vi "Move(SubVI for PI).vi"(5 "Goal":dbl format="%#_13g", 6 "index":i8, 7 "error in":errorcluster) -> (0 "Position After Move":dbl[](array[numeric]) format="%.6f", 3 "error out":errorcluster)   [LabVIEW 2020]
uses:
  Global Parameters.vi
panel:
  out "Position of Global before Move":dbl[](array[numeric])=[95.0] format="%.6f"
  out "Move time":u32
  out "Move+Read Time":u32
  in  "stop":bool
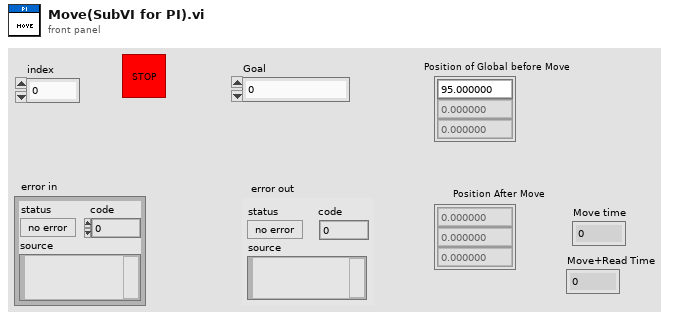
[diagram p1: front panel]
types:
  T1 = enum32{"Bad", "Idle", "Run top level", "Running"}
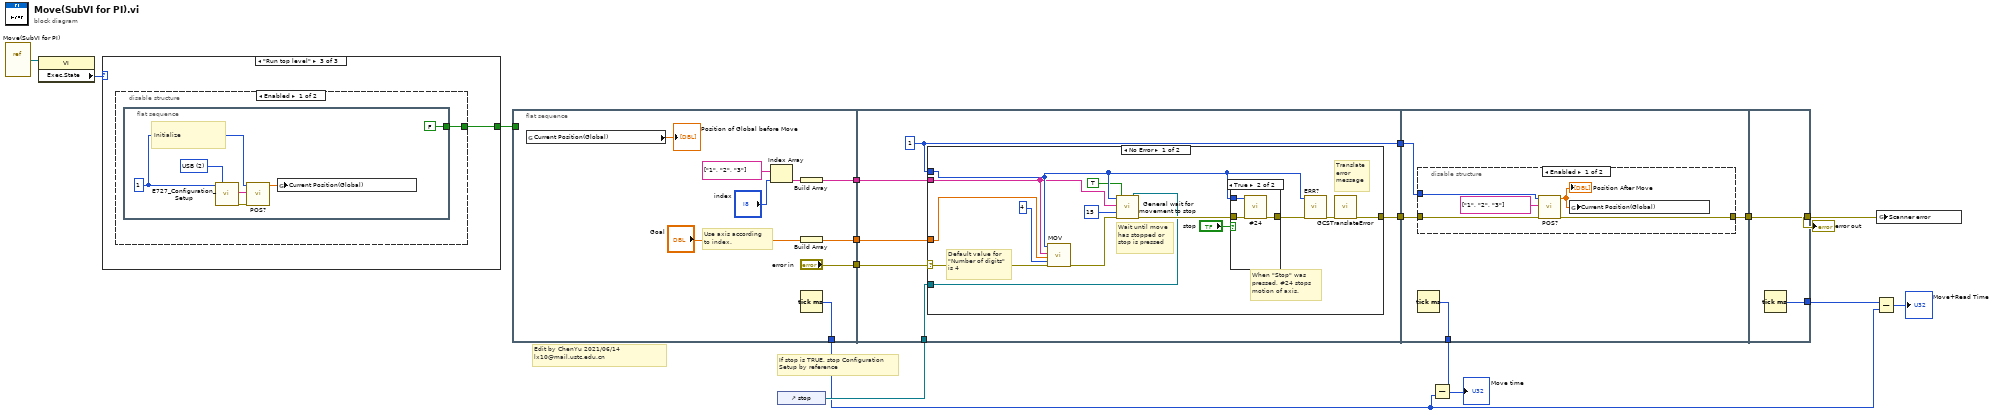
[diagram p0: block diagram]
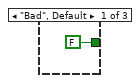
[diagram p2: hidden frame]
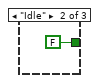
[diagram p3: hidden frame]
diagram:
  # "Edit by ChenYu 2021/06/14 \nlx10@mail.ustc.edu.cn"
  # "If stop is TRUE, stop Configuration\nSetup by reference"
  n1 = vi-ref "Move(SubVI for PI).vi"() -> (w4:refnum<vi>)
  n2 = property class="VI"(reference=w4) -> ("Exec.State"=w5:T1)  [unwired: 1 in, 2 out]
  n3 = case shown="\"Run top level\"" w5 {
    tunnel: [FALSE FALSE w19] -> w6
    frame "Bad", Default {
    }
    frame "Idle" {
    }
    frame "Run top level" {
      n4 = disable-structure shown="Enabled" {
        disable-tunnel: [w20 _] -> w19
        frame Enabled {
          n5 = flat-sequence {
            tunnel: [FALSE] -> w20
            frame #0 {
              w26 = u16 2 items=["RS232", "TCP/IP", "USB"] ("Interface")
              w25 = 1 ("System no.")
              # "Initialize"
              n6 = call "E727_Configuration_Setup.vi"("System no."=w25, "Interface"=w26) -> ("All conn. axes"=w24:string[], "error out"=w22:errorcluster)  [unwired: 12 in, 4 out]
              n7 = call "POS?.vi"("System no."=w25, "Axes to query"=w24, "error in"=w22) -> ("Position"=w23:dbl[])  [unwired: 2 in, 14 out]
              n8 = global write "Global Parameters.vi" "Current Position(Global)"(w23) -> ()
            }
          }
        }
        frame Disabled {
        }
      }
    }
  }
  n9 = flat-sequence {
    tunnel: ["error in"] -> w9
    tunnel: [w31] -> w8
    tunnel: [w30] -> w7
    tunnel: [w32] -> w2
    tunnel: w6 -> [_]
    tunnel: w16 -> [w41]
    tunnel: [w39] -> w15
    tunnel: [w36] -> w14
    tunnel: w7 -> [w40]
    tunnel: w8 -> [w38]
    tunnel: w9 -> [w37]
    tunnel: w15 -> [w62]
    tunnel: w14 -> [w64]
    tunnel: [w61] -> w12
    tunnel: [w63] -> w3
    tunnel: [w71] -> w13
    tunnel: w12 -> [w71]
    tunnel: [w70] -> w10
    frame #0 {
      # "Use axis according\nto index."
      n10 = global read "Global Parameters.vi" "Current Position(Global)"() -> (→"Position of Global before Move":dbl[])
      n11 = Index Array(array=string[] ["1", "2", "3"], index="index") -> (element=w34:string)
      n12 = Build Array(w34) -> (w30:string[])
      n13 = Build Array("Goal") -> (w31:dbl[])
      n14 = Tick Count (ms)() -> (millisecond timer value=w32:u32)
    }
    frame #1 {
      w36 = 1
      n15 = case shown="No Error" w37 {
        selector: w37 -> [w44 w60]
        tunnel: [w55 w60] -> w39
        tunnel: w36 -> [w49 _]
        tunnel: w41 -> [w51 _]
        tunnel: w40 -> [w48 _]
        tunnel: w38 -> [w46 _]
        frame No Error {
          # "When \"Stop\" was \npressed, #24 stops\nmotion of axis."
          # "Translate\nerror \nmessage"
          # "Wait until move\nhas stopped or\nstop is pressed"
          # "Default value for\n\"Number of digits\"\nis 4"
          n16 = call "MOV.vi"("System no."=w49, "Axes to move"=w48, "Position values"=w46, "No.of digits"=i16 4, "error in"=w44) -> ("error out"=w45:errorcluster)  [unwired: 14 out]
          n17 = call "General wait for movement to stop.vi"("System no."=w49, "Axes to wait for"=w48, "Additional wait time, ms"=u32 15, "error in"=w45, "Add. wait only?"=TRUE, "Stop refnum"=w51) -> ("error out"=w54:errorcluster)  [unwired: 2 in, 11 out]
          n18 = case shown="True" "stop" {
            tunnel: w54 -> [w56 w59]
            tunnel: [w56 w58] -> w50
            tunnel: w49 -> [_ w57]
            frame False {
            }
            frame True {
              n19 = call "#24.vi"("System no."=w57, "error in"=w59) -> ("error out"=w58:errorcluster)  [unwired: 17 out]
            }
          }
          n20 = call "ERR?.vi"("System no."=w49, "error in"=w50) -> ("error out"=w52:errorcluster)  [unwired: 17 out]
          n21 = call "GCSTranslateError.vi"("error in"=w52) -> ("error out"=w55:errorcluster)  [unwired: 18 out]
        }
        frame Error {
          # "Error during initialization"
        }
      }
    }
    frame #2 {
      n22 = disable-structure shown="Enabled" {
        disable-tunnel: w64 -> [w68 _]
        disable-tunnel: w62 -> [w66 _]
        disable-tunnel: [w65 _] -> w61
        frame Enabled {
          n23 = call "POS?.vi"("System no."=w68, "Axes to query"=string[] ["1", "2", "3"] ("String"), "error in"=w66) -> ("Position"=w67:dbl[], "error out"=w65:errorcluster)  [unwired: 2 in, 13 out]
          "Position After Move" <- w67
          n24 = global write "Global Parameters.vi" "Current Position(Global)"(w67) -> ()
        }
        frame Disabled {
        }
      }
      n25 = Tick Count (ms)() -> (millisecond timer value=w63:u32)
    }
    frame #3 {
      n26 = Tick Count (ms)() -> (millisecond timer value=w70:u32)
    }
  }
  n27 = control-ref of="stop"() -> (w16:refnum<vi>)
  n28 = Subtract(x=w3, y=w2) -> (x-y=→"Move time":u32)
  n29 = Subtract(x=w10, y=w2) -> (x-y=→"Move+Read Time":u32)
  n30 = global write "Global Parameters.vi" "Scanner error"(w13) -> ()
  "error out" <- w13
